vi "ready_for_imaging.vi"(8 "error in (no error)":errorcluster, 11 "ImagingModeDL100901FlexTrajectory in":refnum<class "ImagingModeDL100901FlexTrajectory.lvclass">) -> (0 "error out":errorcluster, 1 "status out":T1(ring), 2 "ready?":bool, 3 "ImagingModeDL100901FlexTrajectory out":refnum<class "ImagingModeDL100901FlexTrajectory.lvclass">)   [LabVIEW 2010, in "ImagingModeDL100901FlexTrajectory.lvclass"]
uses:
  ImagingModeDL100901FlexTrajectory.lvclass
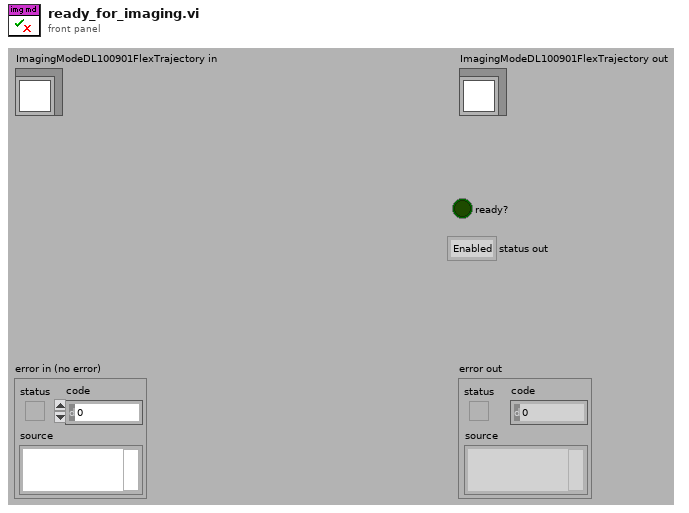
[diagram p1: front panel]
types:
  T1 = enum8{"Enabled", "Disabled", "Disabled and Grayed Out"}
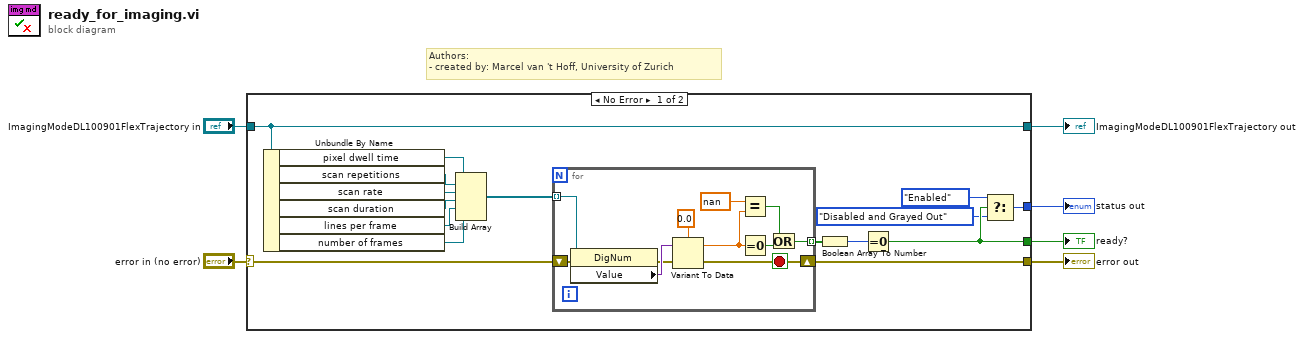
[diagram p0: block diagram]
diagram:
  # "Authors: \n- created by: Marcel van 't Hoff, University of Zurich"
  n1 = case shown="No Error" "error in (no error)" {
    selector: "error in (no error)" -> [w15 w35]
    tunnel: [w12 w35] -> w5
    tunnel: [w11 w34] -> w3
    tunnel: "ImagingModeDL100901FlexTrajectory in" -> [w11 w34]
    tunnel: [w10 _] -> w2
    tunnel: [w7 _] -> w1
    frame No Error {
      n2 = Unbundle By Name(w11) -> ("pixel dwell time"=w22:refnum<vi>, "scan repetitions"=w21:refnum<vi>, "scan rate"=w20:refnum<vi>, "scan duration"=w19:refnum<vi>, "lines per frame"=w18:refnum<vi>, "number of frames"=w17:refnum<vi>)
      n3 = Build Array(w22, w21, w20, w19, w18, w17) -> (w16:refnum<vi>[])
      n4 = for {
        tunnel: w16 -> [w33] mode=indexing
        shift-right: [w23] -> w12
        shift-left: w15 -> [w30]
        tunnel: [w24] -> w14 mode=indexing
        stop <- w23 stop-if-true
        n5 = property class="DigNum"(reference=w33, error in=w30) -> (error out=w29:errorcluster, "Value"=w32:variant)  [unwired: 1 out]
        n6 = Variant To Data(error in=w29, Variant=w32, type=0.0) -> (error out=w23:errorcluster, data=w27:dbl)
        n7 = Equal?(x=nan, y=w27) -> (x = y?=w25:bool)
        n8 = Equal To 0?(x=w27) -> (x = 0?=w26:bool)
        n9 = Or(x=w25, y=w26) -> (x .or. y?=w24:bool)
      }
      n10 = Boolean Array To Number(Boolean array=w14) -> (number=w13:u32)
      n11 = Equal To 0?(x=w13) -> (x = 0?=w10:bool)
      n12 = Select(t=T1."Enabled" ("status"), s=w10, f=T1."Disabled and Grayed Out" ("status")) -> (s? t:f=w7:T1)
    }
    frame Error {
    }
  }
  "error out" <- w5
  "ImagingModeDL100901FlexTrajectory out" <- w3
  "ready?" <- w2
  "status out" <- w1
